vi "OpnCrtRep File.vi"(4 "advisory dialog? (display:T)":bool=TRUE, 5 "file dialog info":T1={"prompt"="", "pattern"="", "default name"="", "start path"=path ""}, 7 "function (open:0)":T4(ring), 8 "error in (not an error)":errorcluster, 9 "deny mode (2)":T2(ring)=enum."deny none", 10 "open mode (0)":T3(ring), 11 "file path":path) -> (0 "error out":errorcluster, 1 "file size (bytes)":i32, 2 "new file path":path, 3 "refnum":refnum<file>)   [LabVIEW 2017, in "NI_FTP.lvlib"]
doc: "This VI is the same as the \"Open/Create/Replace File.vi\" except that it allows you to specify the open and deny modes. It passes the information for the file dialog as a cluster instead of individual parameters.\n\nOpens an existing file, creates a new file, or replaces an existing file, programmatically or interactively using dialog. You can optionally specify a dialog prompt, default file name, start path, or filter pattern, and you can specify open and deny modes when opening a file, plus group and permission when creating a new file. Use this VI with the intermediate Write File+ or Read File+ VIs described below.\n\nfile path is the path name of the file. If file path is empty (default value) or is Not A Path, the VI displays a File dialog box from which you can select a file. Error 43 occurs if the user cancels the dialog. \n\nfunction is the operation to perform:\n\n 0 (open) opens an existing file. Error 7 occurs if the file cannot be found.\n \n 1 (open or create) opens an existing file or creates a new file if one does not exist.\n\n 2 (create or replace) creates a new file or replaces a file if it exists and you give permission. Replacement is done by opening the file and setting EOF to 0. Error 43 occurs if the user elects to disallow the replacement using dialog. \n\n 3 (create) creates a new file. Error 8 occurs if the file already exists.\n\nadvisory dialog? Set TRUE (default) if you want a dialog if function=0 and the file does not exist, or if function=2 or 3 and the file exists.\n\nprompt is the message that appears below the list of files and directories in the file dialog.\n\ndefault name is the initial file name that appears in the selection box of the file dialog.\n\nstart path is the path name to the initially displayed directory in a file dialog. The default value is Not A Path, which is the path to the last directory shown in a file dialog.\n\npattern is the match pattern specification to display only certain types of files or directories. See the description of the File Dialog function for more information.\n\nerror in is a cluster of three elements (error?, code, and source) that describe the upstream error state, that is, the existance of any error preceeding the execution of the VI. The VI executes normally only if no incoming error exists; otherwise it merely passes the error in value to error out. error? is TRUE if an error occurred; the default value is FALSE. code is the error code; the default value is 0. source is in most cases the name of the VI or function that produced the error; the default value is an empty string.\n\nnew file path is the path of the file opened or created. You can use this output to determine the path of a file that you open or create using dialog. new file path returns Not A Path if the user selects Cancel from the dialog box.\n\nrefnum is the reference number of the open file. The value is Not A Refnum if the file cannot be opened.\n\nfile size is the size of the file in bytes; it is also the location of the end of file.\n\nerror out is a cluster of three elements (error?, code, and source) that describe the error state following the execution of the VI. If an incoming error does not exist, the VI executes normally and error out describes the VI's error state; if an incoming error exists, error out equals error in."
uses:
  <vilib>/FTP/NI_FTP.lvlib
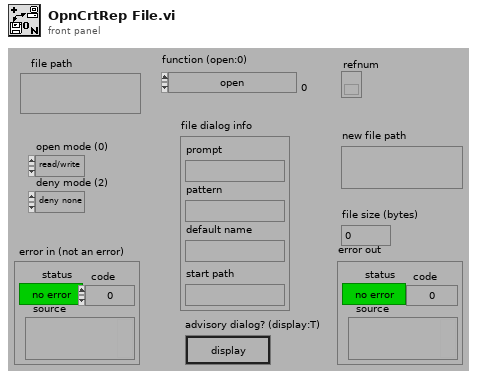
[diagram p1: front panel]
types:
  T1 = cluster{"prompt":string, "pattern":string, "default name":string, "start path":path}
  T2 = enum16{"deny read/write", "deny write-only", "deny none"}
  T3 = enum16{"read/write", "read-only", "write-only", "write-only (truncate)"}
  T4 = enum16{"open", "open or create", "create or replace", "create"}
  T5 = enum16{"open", "replace", "create", "open or create", "replace or create", "replace or create with confirmation"}
  T6 = enum16{"existing file", "new file", "new or existing file", "existing dir", "new dir", "new or existing dir"}[]
  T7 = enum16{"existing file", "new file", "new or existing file", "existing dir", "new dir", "new or existing dir"}
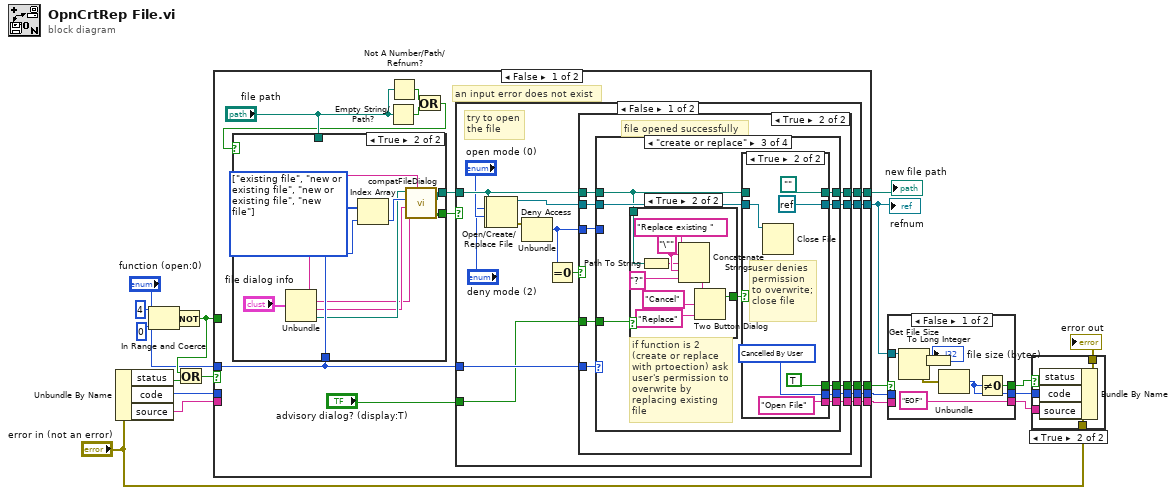
[diagram p0: block diagram]
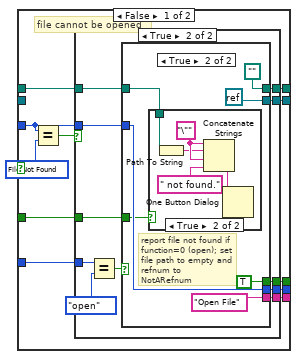
[diagram p4: hidden frame]
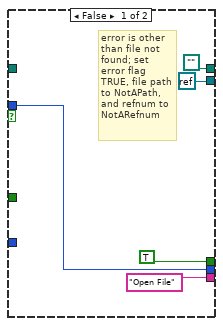
[diagram p5: hidden frame]
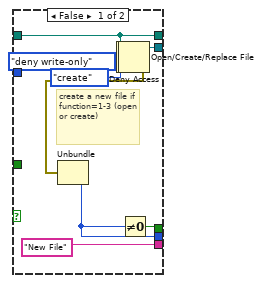
[diagram p6: hidden frame]
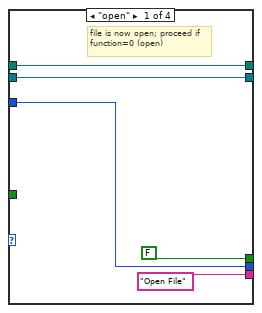
[diagram p8: hidden frame]
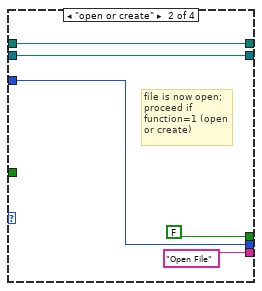
[diagram p9: hidden frame]
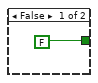
[diagram p10: hidden frame]
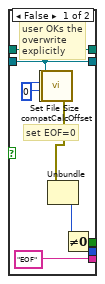
[diagram p11: hidden frame]
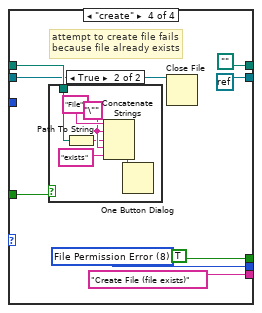
[diagram p12: hidden frame]
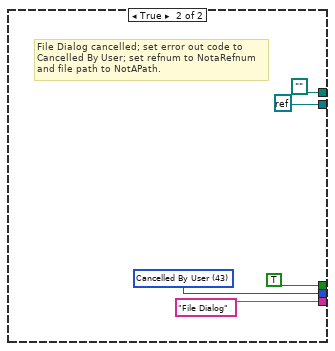
[diagram p14: hidden frame]
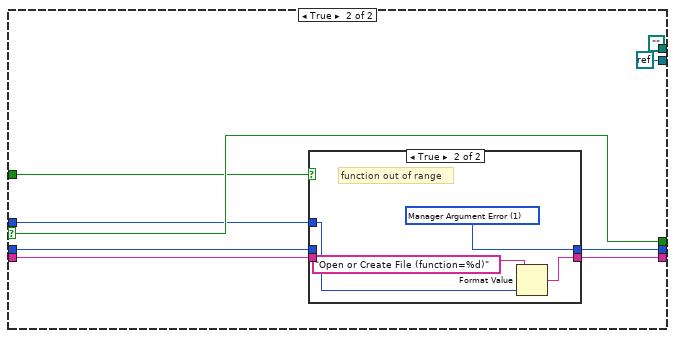
[diagram p16: hidden frame]
diagram:
  n1 = Unbundle By Name("error in (not an error)") -> ("status"=w9:bool, "code"=w8:i32, "source"=w7:string)
  n2 = In Range and Coerce(upper limit=4, x="function (open:0)", lower limit=0) -> (In Range?=w14:bool)  [unwired: 1 out]
  n3 = Not(x=w14) -> (.not. x?=w16:bool)
  n4 = Or(x=w16, y=w9) -> (x .or. y?=w15:bool)
  n5 = case shown="False" w15 {
    selector: w15 -> [_ w190]
    tunnel: [w30 path ""] -> w19
    tunnel: [w29 refnum<k0> refnum] -> w10
    tunnel: [w28 w187] -> w11
    tunnel: [w27 w190] -> w13
    tunnel: [w26 w189] -> w12
    tunnel: w8 -> [_ w188]
    tunnel: w7 -> [_ w186]
    tunnel: "function (open:0)" -> [w20 w185]
    tunnel: w16 -> [_ w184]
    frame False {
      # "an input error does not exist"
      n6 = Empty String/Path?(string/path="file path") -> (empty?=w23:bool)
      n7 = Not A Number/Path/Refnum?(number/path/refnum="file path") -> (NaN/Path/Refnum?=w24:bool)
      n8 = Or(x=w24, y=w23) -> (x .or. y?=w22:bool)
      n9 = case shown="True" w22 {
        selector: w22 -> [w172 _]
        tunnel: [w172 w183] -> w32
        tunnel: [w173 w182] -> w31
        tunnel: "file path" -> [w173 _]
        tunnel: w20 -> [_ w178]
        frame False {
          # "a File Path is supplied (not empty); proceed"
        }
        frame True {
          w179 = T6 [enum."existing file", enum."new or existing file", enum."new or existing file", enum."new file"] items=["existing file", "new file", "new or existing file", "existing dir", "new dir", "new or existing dir"]
          n10 = Unbundle("file dialog info") -> ("prompt"=w181:string, "pattern"=w174:string, "default name"=w175:string, "start path"=w176:path)
          n11 = Index Array(array=w179, index=w178) -> (element=w180:T7)
          n12 = call <vilib>:"compatFileDialog.vi"("prompt"=w181, "pattern"=w174, "default name"=w175, "select mode (2)"=w180, "start path"=w176) -> ("cancelled"=w183:bool, "path"=w182:path)  [unwired: 2 in, 3 out]
        }
      }
      n13 = case shown="False" w32 {
        tunnel: w31 -> [w47 _]
        tunnel: [w46 path ""] -> w30
        tunnel: w20 -> [w45 _]
        tunnel: [w44 refnum<k0> refnum] -> w29
        tunnel: [w42 "File Dialog"] -> w28
        tunnel: [w41 TRUE] -> w27
        tunnel: [w40 w170] -> w26
        tunnel: "advisory dialog? (display:T)" -> [w38 _]
        frame False {
          # "try to open the file"
          n14 = Open/Create/Replace File(file path (use dialog)=w47, access (0:read/write)="open mode (0)") -> (refnum out=w33:refnum<file>, error out=w34:errorcluster)  [unwired: 1 in, 4 out]
          n15 = Deny Access(4:w34, 6:"deny mode (2)", 7:w33) -> (0:w48:errorcluster, 3:w43:refnum<file>)
          n16 = Unbundle(w48) -> ("code"=w37:i32)  [unwired: 2 out]
          n17 = Equal To 0?(x=w37) -> (x = 0?=w39:bool)
          n18 = case shown="True" w39 {
            tunnel: w37 -> [w50 w100]
            tunnel: w47 -> [w57 w106]
            tunnel: [w56 w107] -> w46
            tunnel: w45 -> [w55 w99]
            tunnel: [w54 w105] -> w44
            tunnel: w43 -> [_ w104]
            tunnel: [w53 w103] -> w42
            tunnel: [w52 w102] -> w41
            tunnel: [w51 w101] -> w40
            tunnel: w38 -> [w49 w98]
            frame False {
              w59 = u16 7 items=["No Error", "Manager Argument Error", "Memory Full", "Out of Zone", "End of File", "File Already Open", "Generic File IO Error", "File Not Found", "File Permission Error", "Disk Full", "Duplicate Path", "Too Many Files Open", "Not Enabled", "Resource File Not Found", "Cannot Add Resource", "Resource Not Found", "Image Not Found", "Image Memory Error", "Pen Does Not Exist", "Config Bad Type", "Config Token Not Found", "Config Parse Error", "Config Memory Error", "Bad External Code Format", "Bad External Code Offset", "External Code Not Present", "Null Window", "Destroy Window Mixup", "Null Menu", "Print Aborted", "Bad Print Record", "Print Driver Error", "Windows Error During Print", "Memory Error During Print", "Print Dialog Error", "Generic Print Error", "Invalid Device Refnum", "Device Not Found", "Device Parameter Error", "Device Unit Error", "Can't Open Device", "Device Call Aborted", "Generic Error", "Cancelled By User"]
              # "file cannot be opened"
              n19 = Equal?(x=w50, y=w59) -> (x = y?=w58:bool)
              n20 = case shown="True" w58 {
                tunnel: w57 -> [_ w75]
                tunnel: [path "" w74] -> w56
                tunnel: w55 -> [_ w67]
                tunnel: [refnum<k0> refnum w73] -> w54
                tunnel: ["Open File" w72] -> w53
                tunnel: [TRUE w71] -> w52
                tunnel: [w60 w70] -> w51
                tunnel: w50 -> [w60 w69]
                tunnel: w49 -> [_ w68]
                frame False {
                  # "error is other than file not found; set error flag TRUE, file path to NotAPath, and refnum to NotARefnum"
                }
                frame True {
                  n21 = Equal?(x=w67, y=T4."open") -> (x = y?=w66:bool)
                  n22 = case shown="True" w66 {
                    tunnel: w75 -> [w85 w89]
                    tunnel: [w85 path ""] -> w74
                    tunnel: [w84 refnum<k0> refnum] -> w73
                    tunnel: ["New File" "Open File"] -> w72
                    tunnel: [w83 TRUE] -> w71
                    tunnel: [w80 w90] -> w70
                    tunnel: w69 -> [_ w90]
                    tunnel: w68 -> [_ w86]
                    frame False {
                      # "create a new file if function=1-3 (open or create)"
                      n23 = Open/Create/Replace File(file path (use dialog)=w85, operation (0:open)=T5."create") -> (refnum out=w77:refnum<file>, error out=w78:errorcluster)  [unwired: 1 in, 4 out]
                      n24 = Deny Access(4:w78, 6:T2."deny write-only", 7:w77) -> (0:w82:errorcluster, 3:w84:refnum<file>)
                      n25 = Unbundle(w82) -> ("code"=w80:i32)  [unwired: 2 out]
                      n26 = Not Equal To 0?(x=w80) -> (x != 0?=w83:bool)
                    }
                    frame True {
                      # "report file not found if function=0 (open); set file path to empty and refnum to NotARefnum"
                      n27 = case shown="True" w86 {
                        tunnel: w89 -> [_ w93]
                        frame False {
                        }
                        frame True {
                          w95 = "\""
                          n28 = Path To String(path=w93) -> (string=w94:string)
                          n29 = Concatenate Strings(w95, w94, w95, " not found.") -> (w97:string)
                          n30 = One Button Dialog(message=w97) -> ()  [unwired: 2 out]
                        }
                      }
                    }
                  }
                }
              }
            }
            frame True {
              # "file opened successfully"
              n31 = case shown="\"create or replace\"" w99 {
                tunnel: [w112 w113 w126 path ""] -> w107
                tunnel: w106 -> [w112 w113 w118 w160]
                tunnel: [w111 w114 w125 refnum<k0> refnum] -> w105
                tunnel: w104 -> [w111 w114 w124 w157]
                tunnel: ["Open File" "Open File" w123 "Create File (file exists)"] -> w103
                tunnel: [FALSE FALSE w122 TRUE] -> w102
                tunnel: [w108 w116 w121 w158] -> w101
                tunnel: w100 -> [w108 w116 _ _]
                tunnel: w98 -> [_ _ w119 w159]
                frame "open" {
                  # "file is now open; proceed if function=0 (open)"
                }
                frame "open or create" {
                  # "file is now open; proceed if function=1 (open or create)"
                }
                frame "create or replace" {
                  # "if function is 2 (create or replace with prtoection) ask user's permission to overwrite by replacing existing file"
                  n32 = case shown="True" w119 {
                    tunnel: [FALSE w135] -> w120
                    tunnel: w118 -> [_ w128]
                    frame False {
                    }
                    frame True {
                      w130 = "\""
                      n33 = Path To String(path=w128) -> (string=w129:string)
                      n34 = Concatenate Strings("Replace existing ", w130, w129, w130, "?") -> (w136:string)
                      n35 = Two Button Dialog(message=w136, 1:"Replace", 2:"Cancel") -> (T button?=w135:bool)
                    }
                  }
                  n36 = case shown="True" w120 {
                    tunnel: [w141 path ""] -> w126
                    tunnel: [w146 refnum<k0> refnum] -> w125
                    tunnel: w124 -> [w146 w150]
                    tunnel: ["EOF" "Open File"] -> w123
                    tunnel: [w144 TRUE] -> w122
                    tunnel: [w140 w147] -> w121
                    tunnel: w118 -> [w141 _]
                    frame False {
                      w145 = 0
                      # "set EOF=0"
                      # "user OKs the overwrite explicitly"
                      n37 = call <vilib>:"compatCalcOffset.vi"("pos offset (0)"=w145, "pos mode (0:1)"=w145, "refnum"=w146) -> ("error out"=w139:errorcluster, "offset"=w138:i32, "dup refnum"=w137:refnum<file>)  [unwired: 1 in, 5 out]
                      n38 = Set File Size(4:w139, 6:w138, 7:w137) -> (0:w143:errorcluster)  [unwired: 1 out]
                      n39 = Unbundle(w143) -> ("code"=w140:i32)  [unwired: 2 out]
                      n40 = Not Equal To 0?(x=w140) -> (x != 0?=w144:bool)
                    }
                    frame True {
                      w147 = u16 43 items=["No Error", "Manager Argument Error", "Memory Full", "Out of Zone", "End of File", "File Already Open", "Generic File IO Error", "File Not Found", "File Permission Error", "Disk Full", "Duplicate Path", "Too Many Files Open", "Not Enabled", "Resource File Not Found", "Cannot Add Resource", "Resource Not Found", "Image Not Found", "Image Memory Error", "Pen Does Not Exist", "Config Bad Type", "Config Token Not Found", "Config Parse Error", "Config Memory Error", "Bad External Code Format", "Bad External Code Offset", "External Code Not Present", "Null Window", "Destroy Window Mixup", "Null Menu", "Print Aborted", "Bad Print Record", "Print Driver Error", "Windows Error During Print", "Memory Error During Print", "Print Dialog Error", "Generic Print Error", "Invalid Device Refnum", "Device Not Found", "Device Parameter Error", "Device Unit Error", "Can't Open Device", "Device Call Aborted", "Generic Error", "Cancelled By User"]
                      # "user denies permission to overwrite; close file"
                      n41 = Close File(refnum=w150) -> ()  [unwired: 1 in, 2 out]
                    }
                  }
                }
                frame "create" {
                  w158 = u16 8 items=["No Error", "Argument Error", "Memory Full", "Out of Zone", "End of File", "File Already Open", "Generic File IO Error", "File Not Found", "File Permission Error", "Disk Full", "Duplicate Path", "Too Many Files Open", "Not Enabled", "Resource File Not Found", "Cannot Add Resource", "Resource Not Found", "Image Not Found", "Image Memory Error", "Pen Does Not Exist", "Config Bad Type", "Config Token Not Found", "Config Parse Error", "Config Memory Error", "Bad External Code Format", "Bad External Code Offset", "External Code Not Present", "Null Window", "Destroy Window Mixup", "Null Menu", "Print Aborted", "Bad Print Record", "Print Driver Error", "Windows Error During Print", "Memory Error During Print", "Print Dialog Error", "Generic Print Error", "Invalid Device Refnum", "Device Not Found", "Device Parameter Error", "Device Unit Error", "Can't Open Device", "Device Call Aborted", "Generic Error", "Cancelled By User", "Object ID Too Low", "Object ID Too High", "Object Not In Heap", "Unknown Heap", "Bad DefProc ID", "DefProc Not In Table", "Message Out Of Range", "Null Method", "Unknown Message", "Manager Call Not Supported", "Bad address", "Connection In progress", "Connection timed out", "Connection is already in progress", "Network attribute not supported", "Network error", "Address in use", "System out of memory", "Connection aborted", "Connection refused", "Connection is not connected", "Connection is already connected", "Connection closed", "Initialize error (interapplication manager)", "Bad occurrence", "Wait on unbound occurrence handler", "Occurrence queue overflow", "Bad path", "Semaphore not signaled", "Unrecognized type (interapplication manager)"]
                  # "attempt to create file fails because file already exists"
                  n42 = case shown="True" w159 {
                    tunnel: w160 -> [_ w162]
                    frame False {
                    }
                    frame True {
                      w164 = "\""
                      n43 = Path To String(path=w162) -> (string=w163:string)
                      n44 = Concatenate Strings("File", w164, w163, w164, "exists") -> (w161:string)
                      n45 = One Button Dialog(message=w161) -> ()  [unwired: 2 out]
                    }
                  }
                  n46 = Close File(refnum=w157) -> ()  [unwired: 1 in, 2 out]
                }
              }
            }
          }
        }
        frame True {
          w170 = u16 43 items=["No Error", "Manager Argument Error", "Memory Full", "Out of Zone", "End of File", "File Already Open", "Generic File IO Error", "File Not Found", "File Permission Error", "Disk Full", "Duplicate Path", "Too Many Files Open", "Not Enabled", "Resource File Not Found", "Cannot Add Resource", "Resource Not Found", "Image Not Found", "Image Memory Error", "Pen Does Not Exist", "Config Bad Type", "Config Token Not Found", "Config Parse Error", "Config Memory Error", "Bad External Code Format", "Bad External Code Offset", "External Code Not Present", "Null Window", "Destroy Window Mixup", "Null Menu", "Print Aborted", "Bad Print Record", "Print Driver Error", "Windows Error During Print", "Memory Error During Print", "Print Dialog Error", "Generic Print Error", "Invalid Device Refnum", "Device Not Found", "Device Parameter Error", "Device Unit Error", "Can't Open Device", "Device Call Aborted", "Generic Error", "Cancelled By User"]
          # "File Dialog cancelled; set error out code to Cancelled By User; set refnum to NotaRefnum and file path to NotAPath."
        }
      }
    }
    frame True {
      n47 = case shown="True" w184 {
        tunnel: [w194 w198] -> w189
        tunnel: w188 -> [w194 _]
        tunnel: [w193 w197] -> w187
        tunnel: w186 -> [w193 _]
        tunnel: w185 -> [_ w195]
        frame False {
          # "on an input error, do nothing"
        }
        frame True {
          w198 = u16 1 items=["No Error", "Manager Argument Error", "Memory Full", "Out of Zone", "End of File", "File Already Open", "Generic File IO Error", "File Not Found", "File Permission Error", "Disk Full", "Duplicate Path", "Too Many Files Open", "Not Enabled", "Resource File Not Found", "Cannot Add Resource", "Resource Not Found", "Image Not Found", "Image Memory Error", "Pen Does Not Exist", "Config Bad Type", "Config Token Not Found", "Config Parse Error", "Config Memory Error", "Bad External Code Format", "Bad External Code Offset", "External Code Not Present", "Null Window", "Destroy Window Mixup", "Null Menu", "Print Aborted", "Bad Print Record", "Print Driver Error", "Windows Error During Print", "Memory Error During Print", "Print Dialog Error", "Generic Print Error", "Invalid Device Refnum", "Device Not Found", "Device Parameter Error", "Device Unit Error", "Can't Open Device", "Device Call Aborted", "Generic Error", "Cancelled By User"]
          # "function out of range"
          n48 = Format Value(format string="Open or Create File (function=%d)", value (0)=w195) -> (output string=w197:string)  [unwired: 1 out]
        }
      }
    }
  }
  "new file path" <- w19
  "refnum" <- w10
  n49 = case shown="False" w13 {
    selector: w13 -> [_ w208]
    tunnel: w12 -> [_ w207]
    tunnel: w11 -> [_ w206]
    tunnel: [w204 w208] -> w6
    tunnel: [w201 w207] -> w5
    tunnel: ["EOF" w206] -> w4
    tunnel: w10 -> [w203 _]
    frame False {
      n50 = Get File Size(file=w203) -> (size (in bytes)=w199:i64, 0:w200:errorcluster)  [unwired: 1 in, 1 out]
      n51 = To Long Integer(number=w199) -> (32bit integer=→"file size (bytes)":i32)
      n52 = Unbundle(w200) -> ("code"=w201:i32)  [unwired: 2 out]
      n53 = Not Equal To 0?(x=w201) -> (x != 0?=w204:bool)
    }
    frame True {
    }
  }
  n54 = case shown="True" w6 {
    selector: w6 -> [_ w213]
    tunnel: w5 -> [_ w214]
    tunnel: w4 -> [_ w212]
    tunnel: "error in (not an error)" -> [w209 w211]
    tunnel: [w209 w210] -> w2
    frame False {
    }
    frame True {
      n55 = Bundle By Name(cluster=w211, "status"=w213, "code"=w214, "source"=w212) -> (w210:errorcluster)
    }
  }
  "error out" <- w2
